vi "LJM logger save new program configs.vi"(0 "Working Directory":path, 1 "App name":string="LJM_Exp", 2 "Program Configs":T1={"Data File Prefix"="", "Scan Rate (Hz)"=0.0, "Graph History"=0, "# Channels"=0, "Disable Scaling"=FALSE, "Max File Size (Bytes)"=0, "Channel Setup"={"Name"=["AIN0", "AIN1", "AIN2", "AIN3", "AIN4", "AIN5", "AIN6", "AIN7", "AIN8", "AIN9", "AIN10", "AIN11", "AIN12", "AIN13", "AIN14", "AIN15"], "", "Scaling Equation"=["y=a", "y=b", "y=c", "y=d", "y=e", "y=f", "y=g", "y=h", "y=i", "y=j", "y=k", "y=l", "y=m", "y=n", "y=o", "y=p"], "", "Graph?"=[TRUE, TRUE, TRUE, TRUE, FALSE, FALSE, FALSE, FALSE, FALSE, FALSE, FALSE, FALSE, FALSE, FALSE, FALSE, FALSE]}, "Interval (ms)"=0, "Write To File"=FALSE, "Log Every n Scans"=0}, 5 "error in":errorcluster, 11 "Resolution":u8, 13 "SettlingFactor":u8) -> (14 "Working Directory Out":path, 16 "Program Config Name":string, 19 "error out":errorcluster)   [LabVIEW 2026]
uses:
  Common Logger Controls/Program Config Cluster.ctl
  Common Logger Controls/Channel Setup.ctl
  Instance           1 43Saved   LJM logger save new program configs .vi
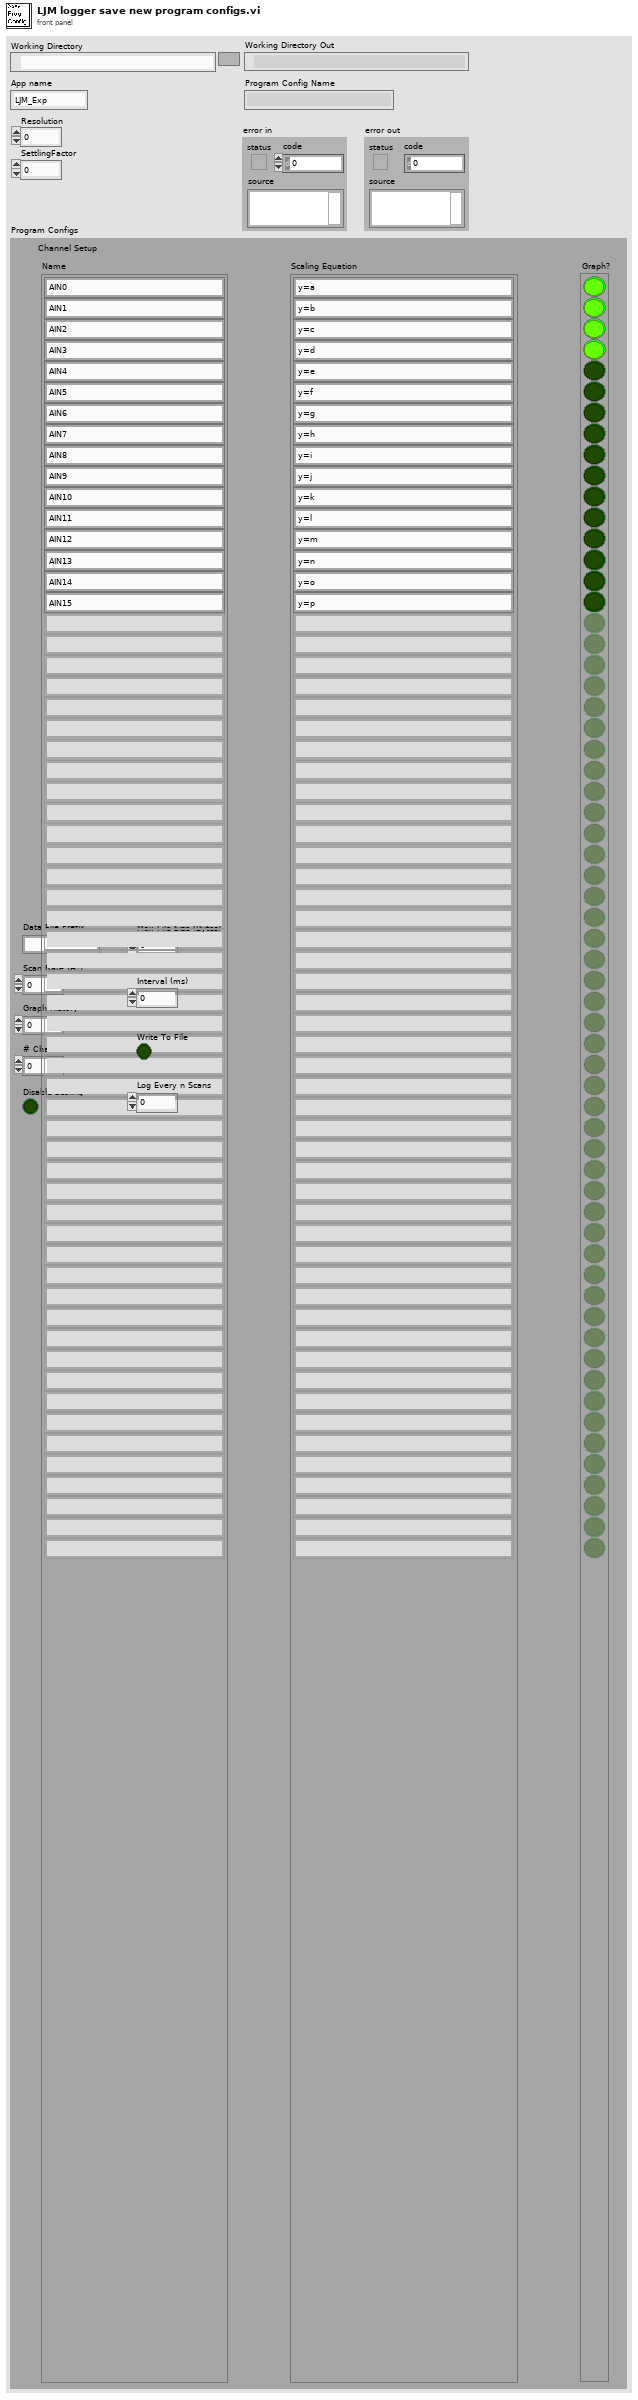
[diagram p1: front panel]
types:
  T1 = typedef "Program Config Cluster.ctl" = cluster{"Data File Prefix":string, "Scan Rate (Hz)":dbl, "Graph History":i32, "# Channels":i32, "Disable Scaling":bool, "Max File Size (Bytes)":i32, "Channel Setup":T2, "Interval (ms)":u32, "Write To File":bool, "Log Every n Scans":i32}
  T2 = typedef "Channel Setup.ctl" = cluster{"Name":string[], string, "Scaling Equation":string[], string, "Graph?":bool[]}
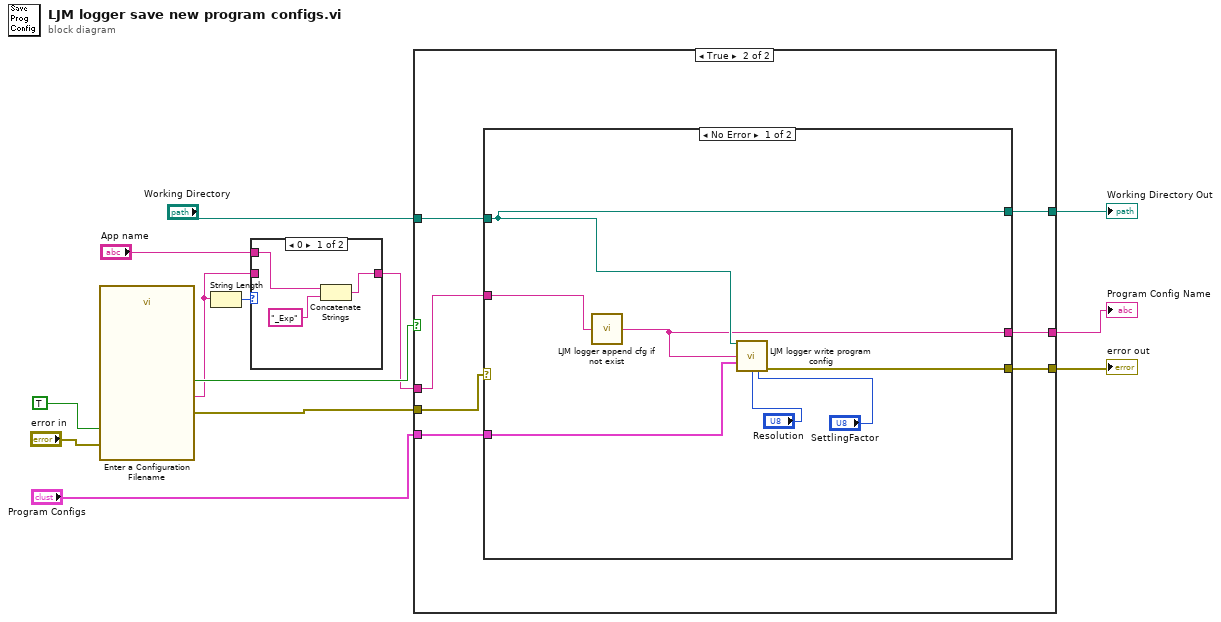
[diagram p0: block diagram]
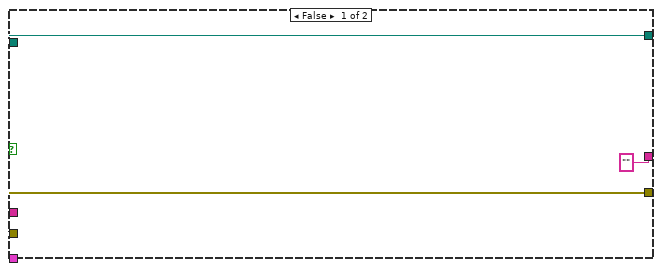
[diagram p3: hidden frame]
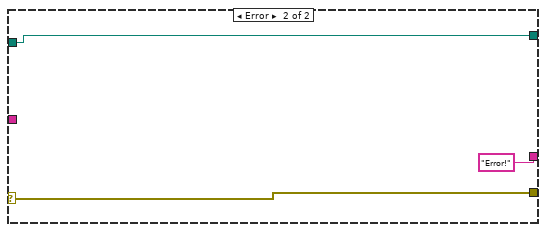
[diagram p4: hidden frame]
diagram:
  n1 = call "Enter a Configuration Filename"("Enable"=TRUE, "error in (no error)"="error in") -> ("Filename"=w6:string, "OK"=w8:bool, "error out"=w9:errorcluster)  [unwired: 15 in]
  n2 = String Length(string=w6) -> (length=w7:i32)
  n3 = case shown="0" w7 {
    tunnel: w6 -> [_ w17]
    tunnel: [w14 w17] -> w5
    tunnel: "App name" -> [w16 _]
    frame 0 {
      n4 = Concatenate Strings(w16, "_Exp" ("string")) -> (w14:string)
    }
    frame 1, Default {
    }
  }
  n5 = case shown="True" w8 {
    tunnel: [w19 w27] -> w13
    tunnel: [w20 w26] -> w4
    tunnel: "Working Directory" -> [w20 w25]
    tunnel: w5 -> [_ w24]
    tunnel: w9 -> [w19 w23]
    tunnel: "Program Configs" -> [_ w22]
    tunnel: ["" ("Output String") w21] -> w2
    frame False {
    }
    frame True {
      n6 = case shown="No Error" w23 {
        selector: w23 -> [_ w37]
        tunnel: [w33 w37] -> w27
        tunnel: [w34 w36] -> w26
        tunnel: w25 -> [w34 w36]
        tunnel: w24 -> [w30 _]
        tunnel: w22 -> [w29 _]
        tunnel: [w28 "Error!" ("Output String")] -> w21
        frame No Error {
          n7 = call "LJM logger append cfg if not exist.vi"("Input String"=w30) -> ("Output String"=w28:string)
          n8 = call "LJM logger write program config.vi"("Working Directory"=w34, "filename"=w28, "Program Configs"=w29, "Resolution"="Resolution", "SettlingFactor"="SettlingFactor") -> ("error out"=w33:errorcluster)  [unwired: 10 in]
        }
        frame Error {
        }
      }
    }
  }
  "error out" <- w13
  "Working Directory Out" <- w4
  "Program Config Name" <- w2
